vi "Mittelwert vorgeben.vi"(11 "Komponente":u16(ring)) -> (3 "Mittelwert":sgl format="%.2f")   [LabVIEW 2020, in "EPA 1065.lvlib" / "HovaCAL Interference verificaton.lvlib"]
uses:
  HovaCAL Interference verificaton.lvlib
  Seiten/FT-IR/FGV FT-IR Aktionen.ctl
  Messdaten/Gewichtung (Stichprobe).ctl
  Messdaten/Aktionen FGV Messdaten.ctl
  Seiten/FT-IR/FT-IR.lvlib
  Messdaten/Messdaten.lvlib
  Seiten/FT-IR/Aktionen EVID-Codes.ctl
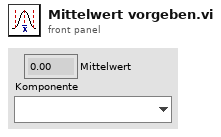
[diagram p1: front panel]
types:
  T1 = typedef "Messdaten.lvlib/Aktionen FGV Messdaten.ctl" = enum16{"lesen", "schreiben", "löschen", "Mittelwerte", "Komponente"}
  T2 = typedef "Messdaten.lvlib/Gewichtung (Stichprobe).ctl" = enum16{"Sample", "Population"}
  T3 = typedef "FT-IR.lvlib/FGV FT-IR Aktionen.ctl" = enum16{"lesen", "NOG setzen", "NOS setzen", "Initialisieren", "speichern", "ALLES setzen", "FT-IR Spektrum loggen", "Komm Stoppen", "Spektrum LogKonfig"}
  T4 = typedef "FT-IR.lvlib/Aktionen EVID-Codes.ctl" = enum16{"lesen", "setzen", "laden", "speichern", "1Hz/5Hz", "Smoothing", "Rolling Average"}
  T5 = typedef "FT-IR.lvlib/1Hz-5Hz Geraet.ctl" = u16
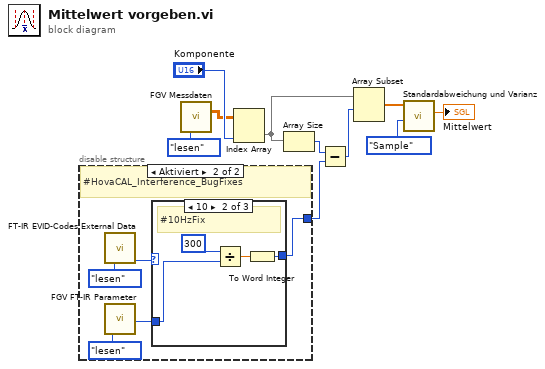
[diagram p0: block diagram]
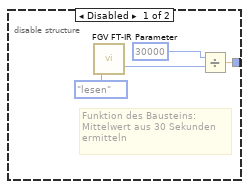
[diagram p2: hidden frame]
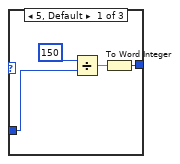
[diagram p3: hidden frame]
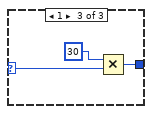
[diagram p4: hidden frame]
diagram:
  n1 = disable-structure shown="Aktiviert" {
    disable-tunnel: [w11 w16] -> w6
    frame Disabled {
      # "Funktion des Bausteins:\nMittelwert aus 30 Sekunden \nermitteln"
      n2 = call "FGV FT-IR Parameter.vi"("Aktion"=FGV_FT-IR_Aktionen."lesen") -> ("Zykluszeit Messdatenverteiler"=w13:u32)  [unwired: 11 in, 7 out]
      n3 = Divide(x=30000, y=w13) -> (x/y=w11:dbl)
    }
    frame Enabled {
      # "#HovaCAL_Interference_BugFixes"
      n4 = call "FT-IR EVID-Codes External Data.vi"("Aktionen"=Aktionen_EVID-Codes."lesen") -> ("1Hz/5Hz Gerät"=w15:T5)  [unwired: 9 in, 5 out]
      n5 = call "FGV FT-IR Parameter.vi"("Aktion"=FGV_FT-IR_Aktionen."lesen") -> ("NoOfScan"=w17:u32)  [unwired: 11 in, 7 out]
      n6 = case shown="10" w15 {
        selector: w15 -> [_ _ w28]
        tunnel: [w20 w24 w29] -> w16
        tunnel: w17 -> [w22 w26 _]
        frame 5, Default {
          n7 = Divide(x=150, y=w22) -> (x/y=w21:dbl)
          n8 = To Word Integer(number=w21) -> (16bit integer=w20:i16)
        }
        frame 10 {
          # "#10HzFix"
          n9 = Divide(x=300, y=w26) -> (x/y=w25:dbl)
          n10 = To Word Integer(number=w25) -> (16bit integer=w24:i16)
        }
        frame 1 {
          n11 = Multiply(x=30, y=w28) -> (x*y=w29:i32)
        }
      }
    }
  }
  n12 = call "FGV Messdaten.vi"("Aktionen"=Aktionen_FGV_Messdaten."lesen") -> ("Messdaten"=w1:sgl[][])  [unwired: 6 in, 8 out]
  n13 = Index Array(array=w1, index (col)="Komponente") -> (element=w2:sgl[])  [unwired: 1 in]
  n14 = Array Size(array=w2) -> (size(s)=w7:i32)
  n15 = Subtract(x=w7, y=w6) -> (x-y=w8:i32)
  n16 = Array Subset(array=w2, index=w8) -> (w5:sgl[])  [unwired: 1 in]
  n17 = call "Standardabweichung und Varianz.vi"("Gewichtung (Stichprobe)"=Gewichtung_(Stichprobe)."Sample", "X"=w5) -> ("Mittelwert"=→"Mittelwert":sgl)  [unwired: 7 in, 2 out]
